vi "Example.vi"   [LabVIEW 2015]
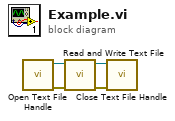
[diagram p0: block diagram]
diagram:
  n1 = call "Open Text File Handle.vi"() -> ("error out"=w3:errorcluster, "Byte Stream File out"=w4:refnum<file>)  [unwired: 10 in]
  n2 = call "Read and Write Text File.vi"("error in (no error)"=w3, "Byte Stream File in"=w4) -> ("error out"=w1:errorcluster, "Byte Stream File out"=w2:refnum<file>)  [unwired: 8 in]
  n3 = call "Close Text File Handle.vi"("error in (no error)"=w1, "Byte Stream File in"=w2) -> ()  [unwired: 10 in]
